vi "Less.vi"() -> ()   [LabVIEW 2017, in "Transparent Assertions.Tests.lvlib" / "Assert Not In Range.lvlib"]
uses:
  Assert Not In Range.lvlib
  src/Transparent Assertions/Transparent Assertions.lvlib
panel:
  out "error out":errorcluster
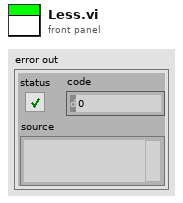
[diagram p1: front panel]
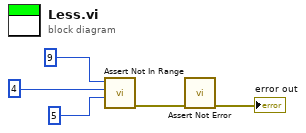
[diagram p0: block diagram]
diagram:
  n1 = call "Assert Not In Range.vi"("Minimum"=5, "Actual"=4, "Maximum"=9) -> ("error out"=w1:errorcluster)  [unwired: 8 in]
  n2 = call "Assert Not Error.vi"("error in (no error)"=w1) -> ("error out"=→"error out":errorcluster)  [unwired: 10 in]
